vi "Eta_Euler2Eta_Quart.vi"(1 "Eta_In":dbl[](array[numeric])) -> (0 "Eta_Out":dbl[](array[numeric]))   [LabVIEW 2011]
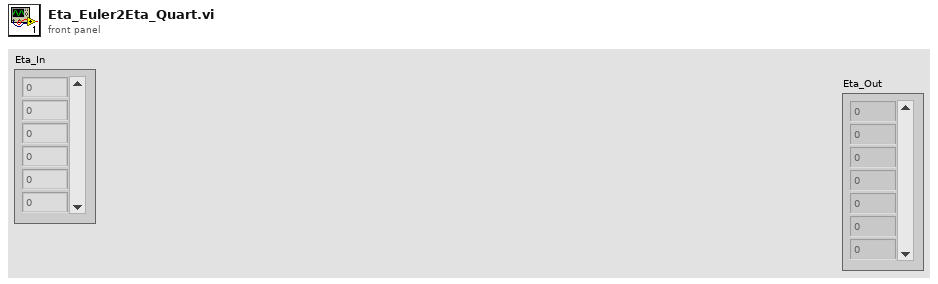
[diagram p1: front panel]
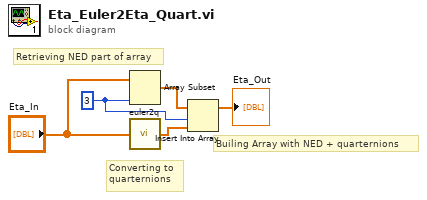
[diagram p0: block diagram]
diagram:
  w2 = 3
  # "Builing Array with NED + quarternions"
  # "Converting to\nquarternions"
  # "Retrieving NED part of array"
  n1 = Array Subset(array="Eta_In", length=w2) -> (w4:dbl[])  [unwired: 1 in]
  n2 = call "euler2q.vi"("Eta"="Eta_In") -> ("q"=w3:dbl[])
  n3 = Insert Into Array(array=w4, index=w2, new element=w3) -> (→"Eta_Out":dbl[])
